vi "2.vi"(11 "文字列入力":string) -> (3 "文字列出力":string)   [LabVIEW 2019]
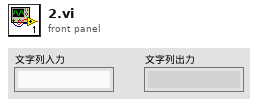
[diagram p1: front panel]
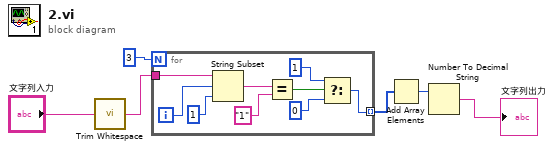
[diagram p0: block diagram]
diagram:
  n1 = call <vilib>:"Trim Whitespace.vi"("string"="文字列入力") -> ("trimmed string"=w2:string)  [unwired: 1 in]
  n2 = for {
    N: 3 -> [_]
    tunnel: w2 -> [w14]
    tunnel: [w7] -> w4 mode=indexing
    i -> [w12]
    n3 = String Subset(string=w14, offset (0)=w12, length (rest)=1) -> (substring=w13:string)
    n4 = Equal?(x=w13, y="1") -> (x = y?=w8:bool)
    n5 = Select(t=1, s=w8, f=0) -> (s? t:f=w7:i32)
  }
  n6 = Add Array Elements(numeric array=w4) -> (sum=w5:i32)
  n7 = Number To Decimal String(number=w5) -> (decimal integer string=→"文字列出力":string)  [unwired: 1 in]
